vi "Chebyshev Order Estimation.vi"(7 "filter type":T3, 8 "error in (no error)":errorcluster, 9 "ripple specs":T1={"passband"=0.1, "stopband"=60.0, "dB/linear? (T: dB)"=TRUE}, 10 "freq specs":T2={"lower pass freq"=0.2, "lower stop freq"=0.3, "higher pass freq"=0.0, "higher stop freq"=0.0}, 11 "sampling freq: fs":dbl=1.0 format="%.2f") -> (0 "error out":errorcluster, 1 "low cutoff freq":dbl, 2 "high cutoff freq":dbl, 3 "estimated order":i32, 4 "passband ripple [dB]":dbl format="%.2f")   [LabVIEW 2020, in "NI_AAL_Filter.lvlib"]
doc: "Estimates the Chebyshev I filter order."
uses:
  <vilib>/Analysis/NI_AAL_Filter.lvlib
  <vilib>/Analysis/3filter.llb/Filter Passband Type.ctl
  <vilib>/Analysis/3filter.llb/Filter Frequence Specification (Design).ctl
  <vilib>/Analysis/3filter.llb/Filter Ripple Specification (Design).ctl
  <vilib>/Analysis/NI_AALBase.lvlib
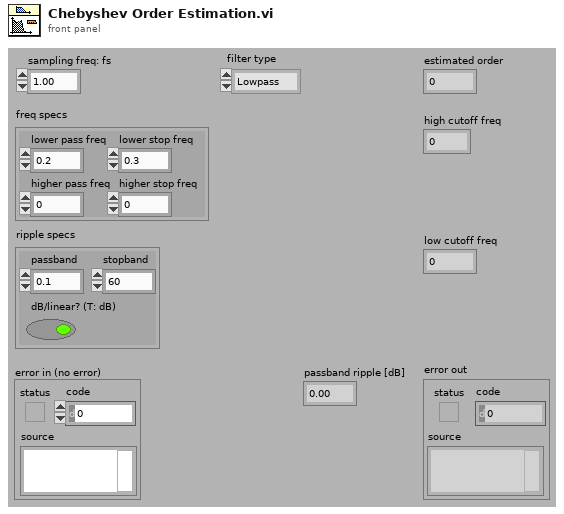
[diagram p1: front panel]
types:
  T1 = typedef "NI_AAL_Filter.lvlib/Filter Ripple Specification (Design).ctl" = cluster{"passband":dbl, "stopband":dbl, "dB/linear? (T: dB)":bool}
  T2 = typedef "NI_AAL_Filter.lvlib/Filter Frequence Specification (Design).ctl" = cluster{"lower pass freq":dbl, "lower stop freq":dbl, "higher pass freq":dbl, "higher stop freq":dbl}
  T3 = typedef "NI_AALBase.lvlib/Filter Passband Type.ctl" = enum32{"Lowpass", "Highpass", "Bandpass", "Bandstop"}
  T4 = enum16{"Butterworth", "Chebyshev", "Inverse Chebyshev", "Elliptic", "Bessel"}
  T5 = cluster{"passband ripple":dbl, "stopband atten":dbl}
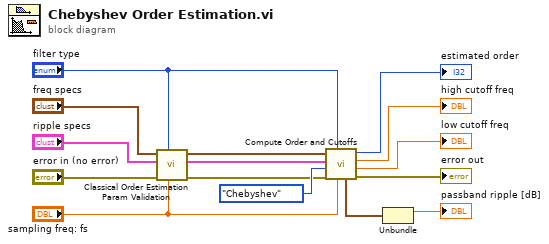
[diagram p0: block diagram]
diagram:
  n1 = call <vilib>:"Classical Order Estimation Param Validation.vi"("fs [Hz]"="sampling freq: fs", "filter type"="filter type", "error in (no error)"="error in (no error)", "ripple specs"="ripple specs", "freq specs [Hz]"="freq specs") -> ("error out"=w8:errorcluster, "dup ripple specs"=w5:T1, "dup freq specs [Hz]"=w6:T2)  [unwired: 1 in, 3 out]
  n2 = call <vilib>:"Compute Order and Cutoffs.vi"("fs [Hz]"="sampling freq: fs", "filter type"="filter type", "error in (no error)"=w8, "design method"=T4."Chebyshev", "ripple specs"=w5, "freq specs [Hz]"=w6) -> ("error out"=→"error out":errorcluster, "low cutoff freq: fl"=→"low cutoff freq":dbl, "high cutoff freq: fh"=→"high cutoff freq":dbl, "n"=→"estimated order":i32, "ripples [dB]"=w4:T5)  [unwired: 1 out]
  n3 = Unbundle(w4) -> ("passband ripple"=→"passband ripple [dB]":dbl)  [unwired: 1 out]
